vi "Finish Scan.vi"(8 "error in (no error)":errorcluster, 11 "Continuous in":refnum<class "Continuous.lvclass">) -> (0 "error out":errorcluster, 3 "Continuous out":refnum<class "Continuous.lvclass">)   [LabVIEW 2009, in "Continuous.lvclass"]
uses:
  Continuous.lvclass
  Instruments/Magnet/Magnet.lvclass
panel:
  out "persis?":bool caption="Persistent"
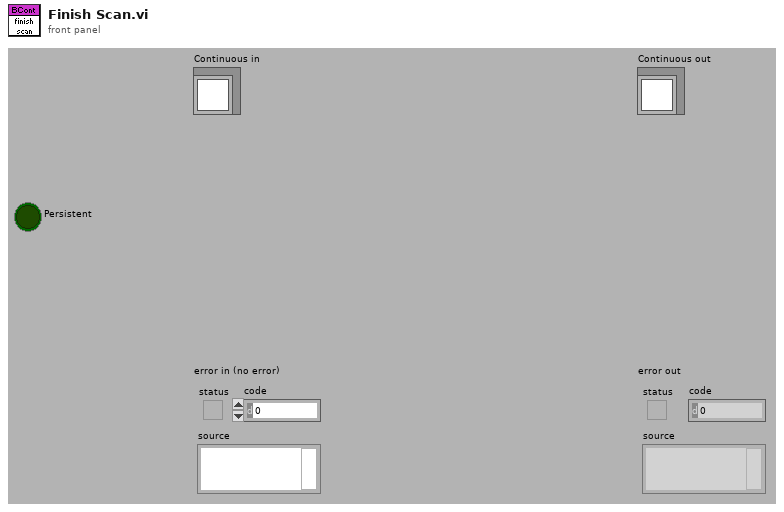
[diagram p1: front panel]
types:
  T1 = typedef "Scanner.lvclass/Range.ctl" = cluster{"xi":dbl, "xf":dbl, "dx":dbl, "Return to...?":bool, "Return to":dbl}
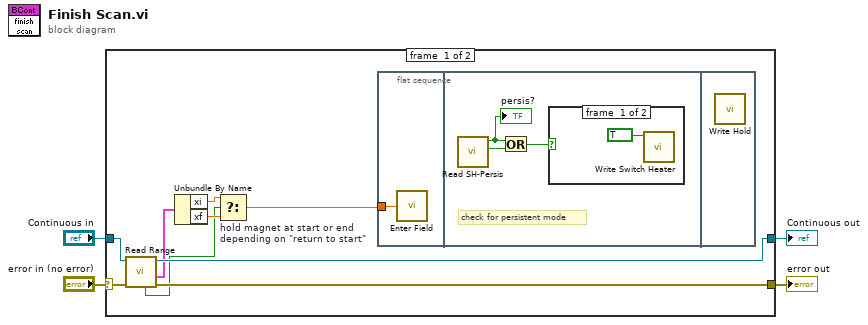
[diagram p0: block diagram]
diagram:
  n1 = case shown="No Error" "error in (no error)" {
    selector: "error in (no error)" -> [w11 w20]
    tunnel: [w13 w20] -> w4
    tunnel: [w12 w19] -> w3
    tunnel: "Continuous in" -> [w10 w19]
    frame #0 {
      n2 = call-dynamic "Read Range.vi"("error in (no error)"=w11, "Scanner.lvclass in"=w10) -> ("error out"=w13:errorcluster, "Range"=w9:T1, "Scanner.lvclass out"=w12:refnum<class "Continuous.lvclass">, "Return to start?"=w6:bool)  [unwired: 6 out]
      n3 = Unbundle By Name(w9) -> ("xi"=w8:dbl, "xf"=w7:dbl)
      n4 = Select "hold magnet at start or end\ndepending on \"return to start\""(t=w8, s=w6, f=w7) -> (s? t:f=w5:dbl)
      n5 = flat-sequence {
        tunnel: w5 -> [w14]
        frame #0 {
          n6 = call "Enter Field.vi"("field"=w14) -> ()  [unwired: 2 in, 3 out]
        }
        frame #1 {
          # "check for persistent mode"
          n7 = call "Read SH-Persis.vi"() -> ("pers?"=w15:bool, "SHon?"=w16:bool)  [unwired: 5 out]
          "persis?" <- w15
          n8 = Or(x=w15, y=w16) -> (x .or. y?=w17:bool)
          n9 = case shown="False" w17 {
            frame #0 {
              n10 = call "Write Switch Heater.vi"("switchheater"=TRUE) -> ()  [unwired: 7 out]
            }
            frame #1 {
            }
          }
        }
        frame #2 {
          n11 = call "Write Hold.vi"() -> ()  [unwired: 8 out]
        }
      }
    }
    frame #1 {
    }
  }
  "error out" <- w4
  "Continuous out" <- w3
